vi "Test MSS Simple.vi"() -> ()   [LabVIEW 2023]
uses:
  Measure and Stimulus Subsystems/Measure and Stimulus Subsystems.lvclass
panel:
  out "error out":errorcluster
  out "Output":variant
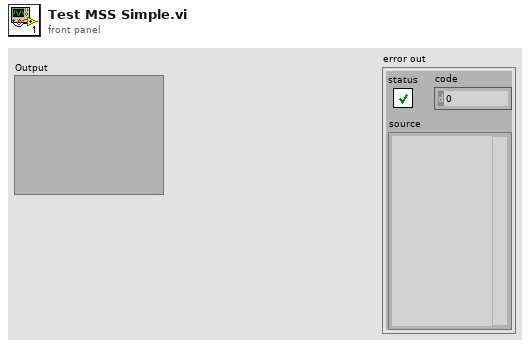
[diagram p1: front panel]
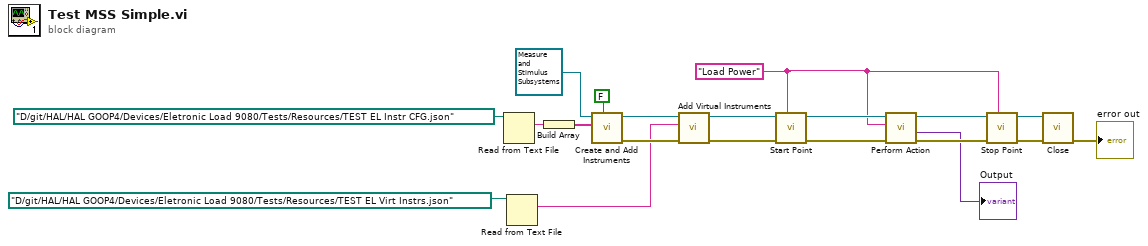
[diagram p0: block diagram]
diagram:
  w2 = "Load Power" ("Task-Point Ident")
  n1 = Read from Text File(file (use dialog)=path "D:/git/HAL/HAL GOOP4/Devices/Eletronic Load 9080/Tests/Resources/TEST EL Instr CFG.json" ("Path")) -> (text=w9:string)  [unwired: 3 in, 3 out]
  n2 = Read from Text File(file (use dialog)=path "D:/git/HAL/HAL GOOP4/Devices/Eletronic Load 9080/Tests/Resources/TEST EL Virt Instrs.json" ("Path")) -> (text=w5:string)  [unwired: 3 in, 3 out]
  n3 = Build Array(w9) -> (w8:string[])
  n4 = call "Create and Add Instruments.vi"("Is Target?"=FALSE, "Physical Intr CFGs"=w8, "MSS in"=refnum<class "Measure and Stimulus Subsystems.lvclass"> refnum) -> ("Error Out"=w19:errorcluster, "MSS out"=w20:refnum<class "Measure and Stimulus Subsystems.lvclass">)  [unwired: 6 in, 1 out]
  n5 = call "Add Virtual Instruments.vi"("error in"=w19, "<JSON CFG>"=w5, "MSS in"=w20) -> ("error out"=w17:errorcluster, "MSS out"=w18:refnum<class "Measure and Stimulus Subsystems.lvclass">)  [unwired: 6 in, 1 out]
  n6 = call "Start Point.vi"("Task-Point Ident"=w2, "error in"=w17, "MSS in"=w18) -> ("error out"=w15:errorcluster, "MSS out"=w16:refnum<class "Measure and Stimulus Subsystems.lvclass">)  [unwired: 7 in]
  n7 = call "Perform Action.vi"("error in"=w15, "Point Ident"=w2, "MSS in"=w16) -> ("error out"=w13:errorcluster, "Output"=→"Output":variant, "MSS out"=w14:refnum<class "Measure and Stimulus Subsystems.lvclass">)  [unwired: 5 in, 1 out]
  n8 = call "Stop Point.vi"("Task-Point Ident"=w2, "error in"=w13, "MSS in"=w14) -> ("error out"=w11:errorcluster, "MSS out"=w12:refnum<class "Measure and Stimulus Subsystems.lvclass">)  [unwired: 7 in]
  n9 = call "Close.vi"("error in"=w11, "MSS in"=w12) -> ("error out"=→"error out":errorcluster)  [unwired: 8 in, 1 out]
